vi "terminate.vi"(0 "reference in":refnum<class "File Controller.lvclass">, 5 "error in (no error)":errorcluster) -> (14 "reference out":refnum<class "File Controller.lvclass">, 19 "error out":errorcluster)   [LabVIEW 2015, in "File Controller.lvclass"]
uses:
  File Controller.lvclass
  APP/excelFile_class/excelFile.lvclass
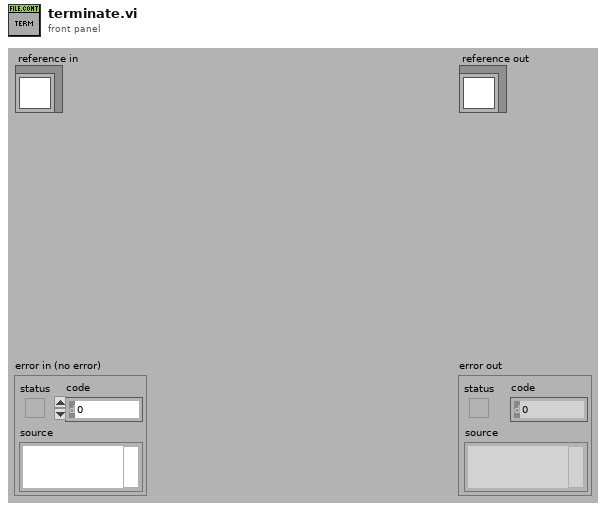
[diagram p1: front panel]
types:
  T1 = typedef "File Controller.lvclass/ObjectAttributesRef.ctl" = refnum<data-value>
  T2 = typedef "File Controller.lvclass/ObjectAttributes.ctl" = cluster{"MyAttribute":dbl, "excelFile_refs":refnum<class "excelFile.lvclass">[], "filePaths":path[], "outlookTemplatePaths":path[], "attachmentTemplatePaths":path[], "configFilePath":path, "not_setting":bool[], "python_ref":refnum<class "python.lvclass">, "TSR":cluster{"number":string, "TSR_path":path, "service_path":path}}
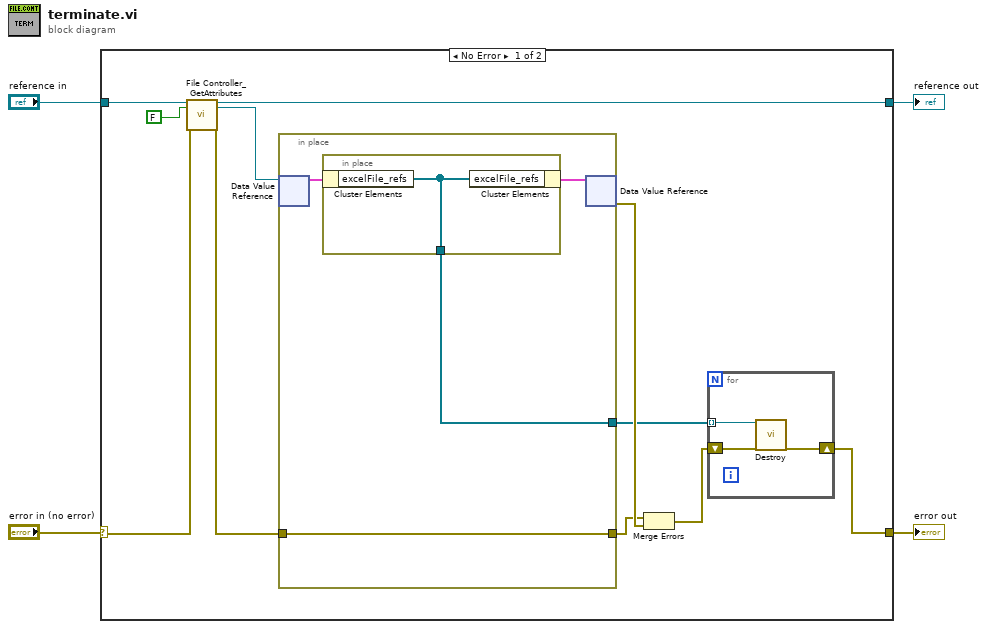
[diagram p0: block diagram]
diagram:
  n1 = case shown="No Error" "error in (no error)" {
    selector: "error in (no error)" -> [w11 w25]
    tunnel: [w5 w25] -> w3
    tunnel: [w9 w24] -> w1
    tunnel: "reference in" -> [w13 w24]
    frame No Error {
      n2 = call "File Controller_GetAttributes.vi"("reference in"=w13, "return data? (T)"=FALSE, "error in (no error)"=w11) -> ("reference out"=w9:refnum<class "File Controller.lvclass">, "attributes ref"=w8:T1, "error out"=w10:errorcluster)  [unwired: 13 in, 1 out]
      n3 = in-place {
        in-place-border: w10 -> [w20]
        in-place-border: [w20] -> w14
        in-place-border: [w19] -> w7
        n4 = in-place-dvr #1(w8) -> (w21:T2)  [unwired: 1 out]
        n5 = in-place {
          in-place-border: [w23] -> w19
          n6 = in-place-cluster #2(w21) -> ("excelFile_refs"=w23:refnum<class "excelFile.lvclass">[])
          n7 = in-place-cluster #2("excelFile_refs"=w23) -> (w22:T2)
        }
        n8 = in-place-dvr #1(w22) -> (w15:errorcluster)  [unwired: 1 out]
      }
      n9 = Merge Errors(w14, w15) -> (w6:errorcluster)
      n10 = for {
        tunnel: w7 -> [w18] mode=indexing
        shift-right: [w16] -> w5
        shift-left: w6 -> [w17]
        n11 = call-dynamic "Destroy.vi"("reference in"=w18, "error in (no error)"=w17) -> ("error out"=w16:errorcluster)  [unwired: 16 in, 1 out]
      }
    }
    frame Error {
    }
  }
  "error out" <- w3
  "reference out" <- w1
